vi "JSON to Elements.vi"(7 "Hierarchy":string[](array[string]), 8 "error in (no error)":errorcluster, 10 "JSON":string) -> (0 "error out":errorcluster, 2 "Elements":T1[](array[typedef]))   [LabVIEW 2020, in "CDM-Config.lvlib" / "Config-JSON.lvclass"]
uses:
  Config-JSON.lvclass
  Config Element.ctl
  Meta Data.ctl
  Value Type.ctl
  32051525-1bd2-438a-8535-b47acd83b430.vi
  a4bd2cb9-4341-4b33-9b2d-4e8a11acea42.vi
  7caed5f1-afa0-46fa-a851-49cc2cde967f.vi
  5cc5a0b3-4775-4e46-a41f-c24ffc72b951.vi
  <vilib>/JDP Science/JSONtext/JSON text to Variant.vi
  <vilib>/JDP Science/JSONtext/LVClass Serializer/JSONtext LVClass Serializer.lvclass
  Config-JSON.lvclass/Config-JSON.ctl
  <vilib>/JDP Science/JSONtext/JSONtext.lvlib
  CDM-Config.lvlib
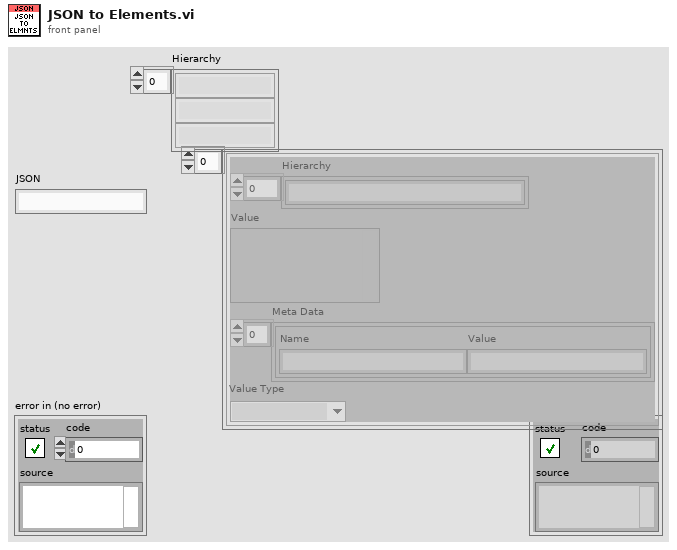
[diagram p1: front panel]
types:
  T1 = typedef "CDM-Config.lvlib/Config Element.ctl" = cluster{"Hierarchy":string[], "Value":variant, "Meta Data":T2[], "Value Type":T3}
  T2 = typedef "CDM-Config.lvlib/Meta Data.ctl" = cluster{"Name":string, "Value":string}
  T3 = typedef "CDM-Config.lvlib/Value Type.ctl" = enum16{"String", "Number", "Bool", "Object", "Array"}
  T4 = typedef "JSONtext.lvlib/JSON Value Type.ctl" = enum16{"Not a JSON Value", "JSON Object", "JSON Array", "String", "Number", "true", "false", "null"}
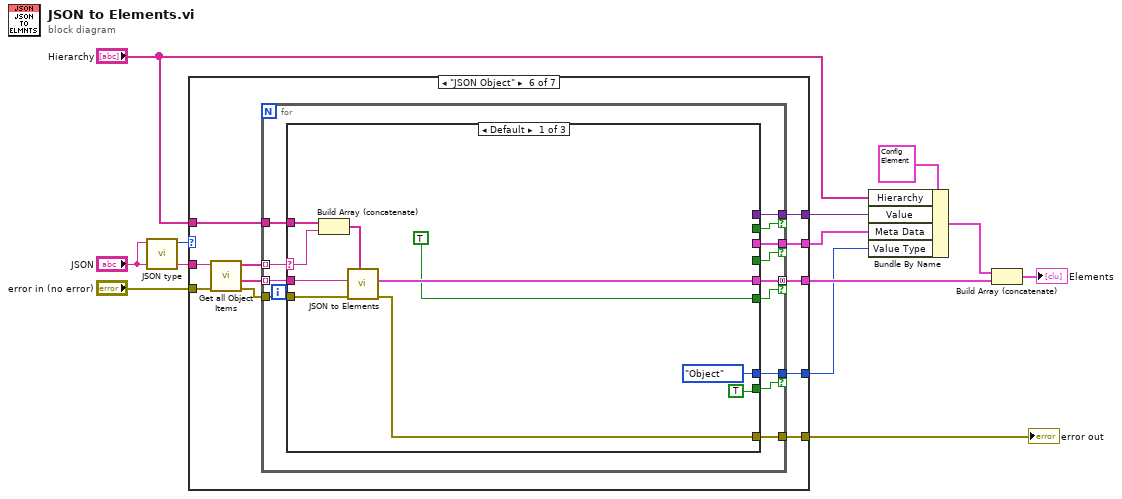
[diagram p0: block diagram]
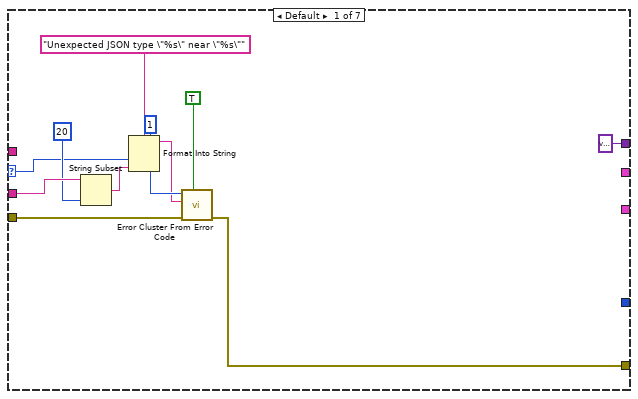
[diagram p2: hidden frame]
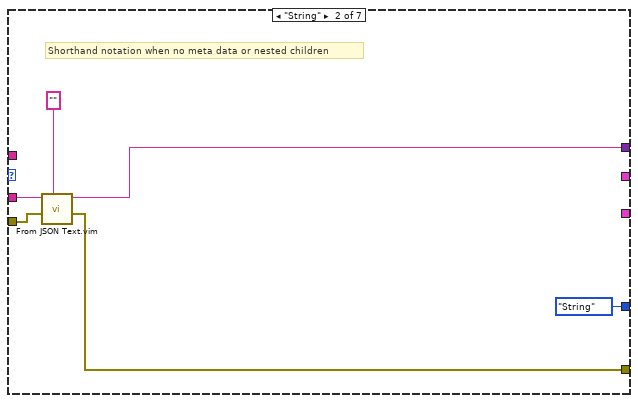
[diagram p3: hidden frame]
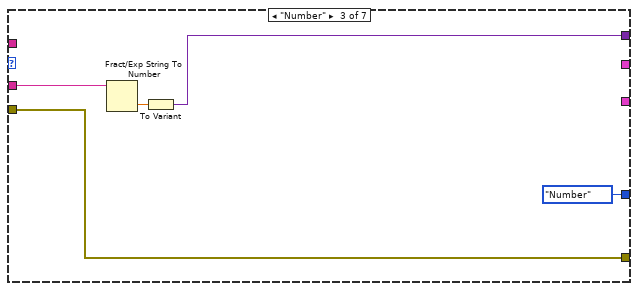
[diagram p4: hidden frame]
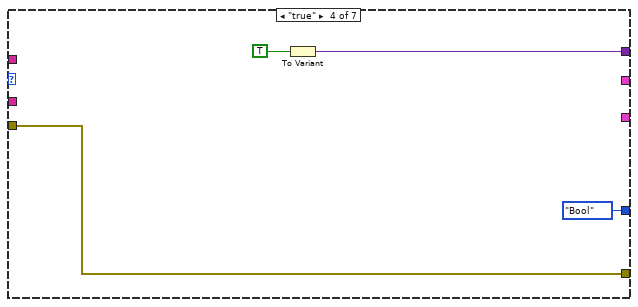
[diagram p5: hidden frame]
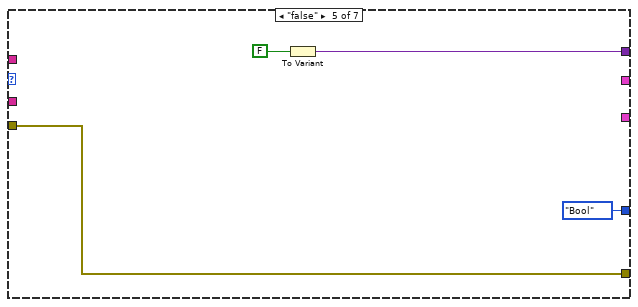
[diagram p6: hidden frame]
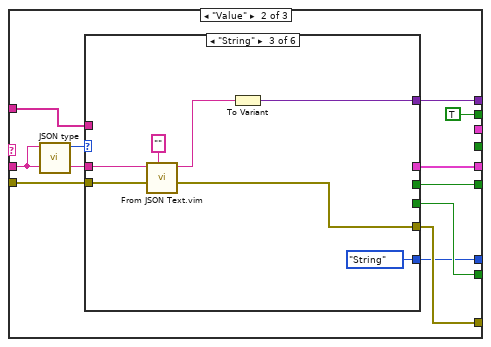
[diagram p7: hidden frame]
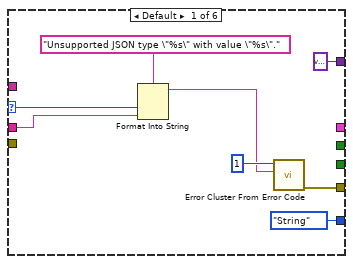
[diagram p8: hidden frame]
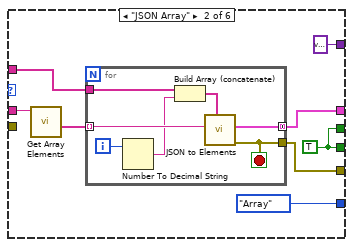
[diagram p9: hidden frame]
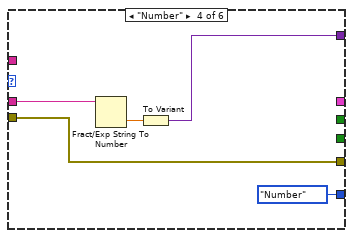
[diagram p10: hidden frame]
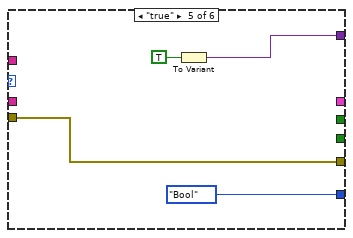
[diagram p11: hidden frame]
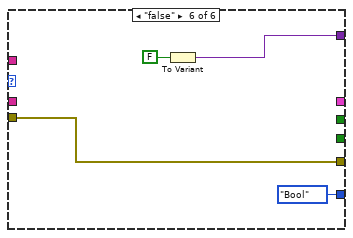
[diagram p12: hidden frame]
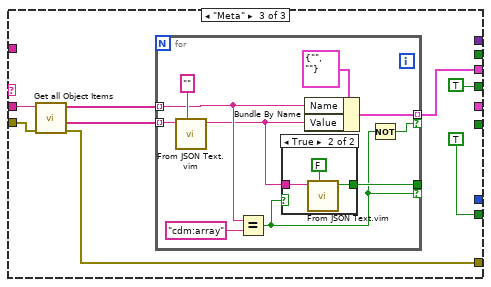
[diagram p13: hidden frame]
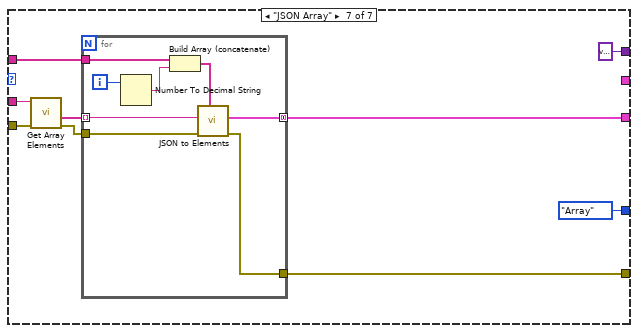
[diagram p15: hidden frame]
diagram:
  n1 = call <vilib>:"JSON type.vi"("JSON"="JSON") -> ("JSON Value Type"=w9:T4)  [unwired: 9 in, 1 out]
  n2 = case shown="\"JSON Object\"" w9 {
    selector: w9 -> [w16 _ _ _ _ _ _]
    tunnel: "error in (no error)" -> [w23 w28 w34 w36 w40 w53 w160]
    tunnel: [_ _ _ _ _ w48 _] -> w5
    tunnel: "Hierarchy" -> [_ _ _ _ _ w47 w157]
    tunnel: [_ _ _ _ _ w46 w156] -> w11
    tunnel: [w14 w27 w34 w36 w40 w45 w155] -> w8
    tunnel: "JSON" -> [w19 w29 w33 _ _ w44 w154]
    tunnel: [_ Value_Type."String" ("Value Type") Value_Type."Number" ("Value Type") Value_Type."Bool" ("Value Type") Value_Type."Bool" ("Value Type") w43 Value_Type."Array" ("Value Type")] -> w2
    tunnel: [variant ("Variant") w25 w31 w37 w41 w49 variant ("Variant")] -> w1
    frame Default {
      n3 = String Subset(string=w19, length (rest)=20 ("length (rest)")) -> (substring=w17:string)  [unwired: 1 in]
      n4 = Format Into String(format string="Unexpected JSON type \"%s\" near \"%s\"", w16, w17) -> (resulting string=w15:string)  [unwired: 2 in, 1 out]
      n5 = call <vilib>:"Error Cluster From Error Code.vi"("show call chain? (False)"=TRUE, "error in (no error)"=w23, "error message (\"\")"=w15, "error code (0)"=1) -> ("error out"=w14:errorcluster)  [unwired: 5 in]
    }
    frame "String" {
      # "Shorthand notation when no meta data or nested children"
      n6 = call "From JSON Text.vim"("Data Type and Default Value"="", "error in (no error)"=w28, "JSON"=w29) -> ("error out"=w27:errorcluster, "Data out"=w25:string)  [unwired: 7 in]
    }
    frame "Number" {
      n7 = Fract/Exp String To Number(string=w33) -> (number=w32:dbl)  [unwired: 3 in, 1 out]
      n8 = To Variant(anything=w32) -> (Variant=w31:variant)
    }
    frame "true" {
      n9 = To Variant(anything=TRUE) -> (Variant=w37:variant)
    }
    frame "false" {
      n10 = To Variant(anything=FALSE) -> (Variant=w41:variant)
    }
    frame "JSON Object" {
      n11 = call <vilib>:"Get all Object Items.vi"("error in (no error)"=w53, "JSON"=w44) -> ("error out"=w50:errorcluster, "<JSON>"=w51:string[], "Item Names"=w52:string[])  [unwired: 6 in, 1 out]
      n12 = for {
        tunnel: w52 -> [w66] mode=indexing
        tunnel: w51 -> [w65] mode=indexing
        tunnel: w50 -> [w64]
        tunnel: w47 -> [w63]
        tunnel: [w62] -> w48 if=w61
        tunnel: [w60] -> w49 if=w55
        tunnel: [w59] -> w46 mode=concatenating if=w57
        tunnel: [w58] -> w45
        tunnel: [w54] -> w43 if=w56
        n13 = case shown="Default" w66 {
          selector: w66 -> [w75 _ _]
          tunnel: w65 -> [w73 w83 w136]
          tunnel: w64 -> [w72 w85 w135]
          tunnel: w63 -> [w76 w80 _]
          tunnel: [_ _ w138] -> w62
          tunnel: [_ _ TRUE] -> w61
          tunnel: [_ w87 _] -> w60
          tunnel: [_ TRUE _] -> w55
          tunnel: [w71 w79 _] -> w59
          tunnel: [w70 w84 w132] -> w58
          tunnel: [TRUE w78 _] -> w57
          tunnel: [TRUE w81 TRUE] -> w56
          tunnel: [Value_Type."Object" ("Value Type") w77 _] -> w54
          frame Default {
            n14 = Build Array (concatenate)(w76, w75) -> (w74:string[])
            n15 = call "JSON to Elements.vi"("Hierarchy"=w74, "error in (no error)"=w72, "JSON"=w73) -> ("error out"=w70:errorcluster, "Elements"=w71:T1[])  [unwired: 7 in]
          }
          frame "Value" {
            n16 = call <vilib>:"JSON type.vi"("JSON"=w83) -> ("JSON Value Type"=w82:T4)  [unwired: 9 in, 1 out]
            n17 = case shown="\"String\"" w82 {
              selector: w82 -> [w90 _ _ _ _ _]
              tunnel: [variant ("Variant") variant ("Variant") w111 w118 w125 w129] -> w87
              tunnel: w85 -> [_ _ w115 w121 w123 w127]
              tunnel: [w95 w98 w114 w121 w123 w127] -> w84
              tunnel: w83 -> [w89 w103 w113 w122 _ _]
              tunnel: [_ w99 _ _ _ _] -> w81
              tunnel: w80 -> [_ w101 _ _ _ _]
              tunnel: [_ w100 _ _ _ _] -> w79
              tunnel: [_ w99 _ _ _ _] -> w78
              tunnel: [Value_Type."String" ("Value Type") Value_Type."Array" ("Value Type") Value_Type."String" ("Value Type") Value_Type."Number" ("Value Type") Value_Type."Bool" ("Value Type") Value_Type."Bool" ("Value Type")] -> w77
              frame Default {
                n18 = Format Into String(format string="Unsupported JSON type \"%s\" with value \"%s\".", w90, w89) -> (resulting string=w88:string)  [unwired: 2 in, 1 out]
                n19 = call <vilib>:"Error Cluster From Error Code.vi"("error message (\"\")"=w88, "error code (0)"=1) -> ("error out"=w95:errorcluster)  [unwired: 7 in]
              }
              frame "JSON Array" {
                w99 = TRUE
                n20 = call <vilib>:"Get Array Elements.vi"("JSON"=w103) -> ("<JSON>"=w102:string[])  [unwired: 8 in, 2 out]
                n21 = for {
                  tunnel: w102 -> [w110] mode=indexing
                  tunnel: w101 -> [w108]
                  tunnel: [w105] -> w100 mode=concatenating
                  tunnel: [w104] -> w98
                  i -> [w107]
                  stop <- w104 stop-if-true
                  n22 = Number To Decimal String(number=w107) -> (decimal integer string=w106:string)  [unwired: 1 in]
                  n23 = Build Array (concatenate)(w108, w106) -> (w109:string[])
                  n24 = call "JSON to Elements.vi"("Hierarchy"=w109, "JSON"=w110) -> ("error out"=w104:errorcluster, "Elements"=w105:T1[])  [unwired: 8 in]
                }
              }
              frame "String" {
                n25 = call "From JSON Text.vim"("Data Type and Default Value"="", "error in (no error)"=w115, "JSON"=w113) -> ("error out"=w114:errorcluster, "Data out"=w116:string)  [unwired: 7 in]
                n26 = To Variant(anything=w116) -> (Variant=w111:variant)
              }
              frame "Number" {
                n27 = Fract/Exp String To Number(string=w122) -> (number=w119:dbl)  [unwired: 3 in, 1 out]
                n28 = To Variant(anything=w119) -> (Variant=w118:variant)
              }
              frame "true" {
                n29 = To Variant(anything=TRUE) -> (Variant=w125:variant)
              }
              frame "false" {
                n30 = To Variant(anything=FALSE) -> (Variant=w129:variant)
              }
            }
          }
          frame "Meta" {
            n31 = call <vilib>:"Get all Object Items.vi"("error in (no error)"=w135, "JSON"=w136) -> ("error out"=w132:errorcluster, "<JSON>"=w134:string[], "Item Names"=w133:string[])  [unwired: 6 in, 1 out]
            n32 = for {
              tunnel: w134 -> [w148] mode=indexing
              tunnel: w133 -> [w144] mode=indexing
              tunnel: [w145] -> w138 mode=indexing if=w141
              tunnel: [w140] -> _ if=w139
              n33 = call "From JSON Text.vim"("Data Type and Default Value"="", "JSON"=w148) -> ("Data out"=w142:string)  [unwired: 8 in, 1 out]
              n34 = Equal?(x=w144, y="cdm:array") -> (x = y?=w139:bool)
              n35 = case shown="True" w139 {
                tunnel: w142 -> [_ w151]
                tunnel: [_ w149] -> w140
                frame False {
                }
                frame True {
                  n36 = call "From JSON Text.vim"("Data Type and Default Value"=FALSE, "JSON"=w151) -> ("Data out"=w149:bool)  [unwired: 8 in, 1 out]
                }
              }
              n37 = Bundle By Name(cluster=T2 {"Name"="", "Value"=""} ("Meta Data"), "Name"=w144, "Value"=w142) -> (w145:T2)
              n38 = Not(x=w139) -> (.not. x?=w141:bool)
            }
          }
        }
      }
    }
    frame "JSON Array" {
      n39 = call <vilib>:"Get Array Elements.vi"("error in (no error)"=w160, "JSON"=w154) -> ("error out"=w158:errorcluster, "<JSON>"=w159:string[])  [unwired: 7 in, 1 out]
      n40 = for {
        tunnel: w159 -> [w168] mode=indexing
        tunnel: w158 -> [w167]
        tunnel: w157 -> [w166]
        tunnel: [w165] -> w156 mode=concatenating
        tunnel: [w164] -> w155
        i -> [w162]
        n41 = Number To Decimal String(number=w162) -> (decimal integer string=w161:string)  [unwired: 1 in]
        n42 = Build Array (concatenate)(w166, w161) -> (w163:string[])
        n43 = call "JSON to Elements.vi"("Hierarchy"=w163, "error in (no error)"=w167, "JSON"=w168) -> ("error out"=w164:errorcluster, "Elements"=w165:T1[])  [unwired: 7 in]
      }
    }
  }
  "error out" <- w8
  n44 = Bundle By Name(cluster=T1 {"Hierarchy"=[], "Value"=variant(string ""), "Meta Data"=[], "Value Type"=enum."String"} ("Config Element"), "Hierarchy"="Hierarchy", "Value"=w1, "Meta Data"=w5, "Value Type"=w2) -> (w4:T1)
  n45 = Build Array (concatenate)(w4, w11) -> (→"Elements":T1[])
